vi "find same SplitMode number for traverse.vi"(8 "error in (no error)":errorcluster caption="错误输入（无错误）", 10 "Data in":cluster{"Split Mode":i32, "#sameMode":i32}={"Split Mode"=-1, "#sameMode"=0}, 11 "Class in":refnum<class "PanelRootNode.lvclass"> caption="DNL_LabVIEW Object in") -> (0 "error out":errorcluster caption="错误输出", 2 "Data out":cluster{"Split Mode":i32, "#sameMode":i32}, 3 "Class out":refnum<class "PanelRootNode.lvclass"> caption="DNL_LabVIEW Object out", 4 "Stop Traverse":bool)   [LabVIEW 2013, in "PanelRootNode.lvclass"]
uses:
  PanelRootNode.lvclass
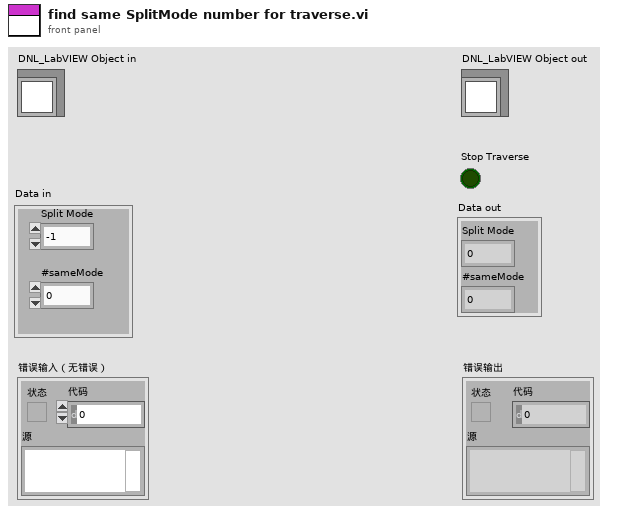
[diagram p1: front panel]
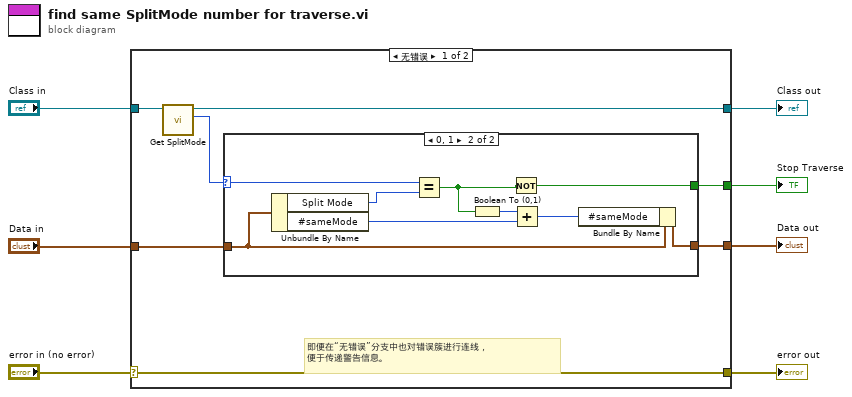
[diagram p0: block diagram]
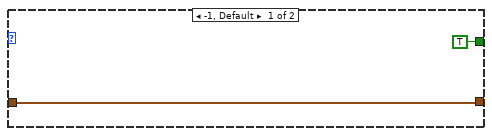
[diagram p2: hidden frame]
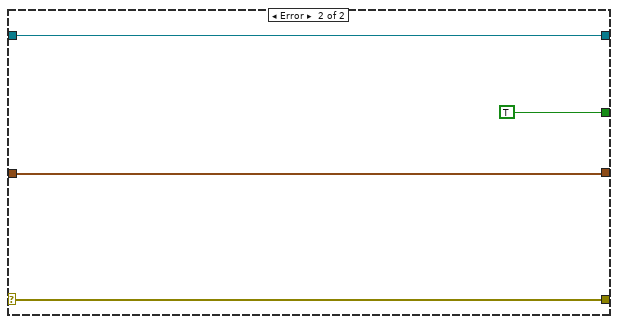
[diagram p3: hidden frame]
diagram:
  n1 = case shown="无错误" "error in (no error)" {
    selector: "error in (no error)" -> [w14 w29]
    tunnel: [w14 w29] -> w6
    tunnel: [w12 w28] -> w4
    tunnel: "Class in" -> [w13 w28]
    tunnel: "Data in" -> [w11 w27]
    tunnel: [w10 w27] -> w2
    tunnel: [w8 TRUE] -> w1
    frame No Error {
      # "即便在“无错误”分支中也对错误簇进行连线，\n便于传递警告信息。"
      n2 = call-dynamic "Get SplitMode.vi"("PanelDataNode 输入"=w13) -> ("Split Mode"=w9:i32, "PanelDataNode 输出"=w12:refnum<class "PanelRootNode.lvclass">)  [unwired: 8 in, 1 out]
      n3 = case shown="0, 1" w9 {
        selector: w9 -> [_ w19]
        tunnel: w11 -> [w16 w22]
        tunnel: [w16 w20] -> w10
        tunnel: [TRUE w17] -> w8
        frame -1, Default {
        }
        frame 0, 1 {
          n4 = Unbundle By Name(w22) -> ("Split Mode"=w25:i32, "#sameMode"=w23:i32)
          n5 = Equal?(x=w19, y=w25) -> (x = y?=w18:bool)
          n6 = Boolean To (0,1)(Boolean=w18) -> (0, 1=w24:i16)
          n7 = Not(x=w18) -> (.not. x?=w17:bool)
          n8 = Add(x=w24, y=w23) -> (x+y=w21:i32)
          n9 = Bundle By Name(cluster=w22, "#sameMode"=w21) -> (w20:cluster{"Split Mode":i32, "#sameMode":i32})
        }
      }
    }
    frame Error {
    }
  }
  "error out" <- w6
  "Class out" <- w4
  "Data out" <- w2
  "Stop Traverse" <- w1
